vi "HideHistoryGraph.vi"(8 "error in":errorcluster caption="错误输入（无错误）", 11 "PCM MenuVIPanelSplit.lvclass":refnum<class "PCM MenuVIPanelSplit.lvclass">) -> (0 "error out":errorcluster caption="错误输出", 3 "PCM MenuVIPanelSplit.lvclass out":refnum<class "PCM MenuVIPanelSplit.lvclass">)   [LabVIEW 2016, in "PCM MenuVIPanelSplit.lvclass"]
uses:
  PCM MenuVIPanelSplit.lvclass
  C:/Users/CL/Desktop/ZcDAQprj0811/ZcDAQprj/Modules/DAQ-Display/PanelSplitToolkit/PanelRootNode/PanelRootNode.lvclass
  PanelSplitToolkit/PanelRootNode/PanelRootNode.lvclass
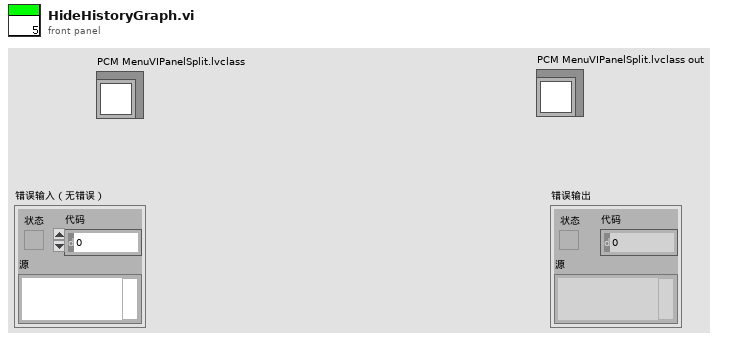
[diagram p1: front panel]
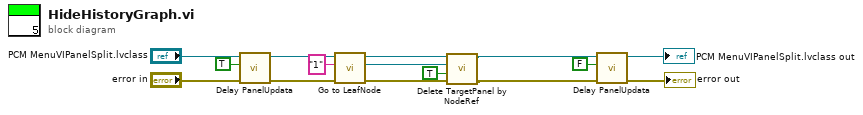
[diagram p0: block diagram]
diagram:
  n1 = call "Delay PanelUpdata.vi"("error in"="error in", "延迟前面板更新"=TRUE, "PanelRootNode 输入"="PCM MenuVIPanelSplit.lvclass") -> ("error out"=w13:errorcluster, "PanelRootNode 输出"=w11:refnum<class "PCM MenuVIPanelSplit.lvclass">)  [unwired: 7 in]
  n2 = call-dynamic "Go to LeafNode.vi"("error in"=w13, "LeafNumber"="1", "PanelRootNode 输入"=w11) -> ("error out"=w4:errorcluster, "Node*"=w2:refnum<data-value>, "PanelRootNode 输出"=w6:refnum<class "PCM MenuVIPanelSplit.lvclass">)  [unwired: 5 in, 1 out]
  n3 = call-dynamic "Delete TargetPanel by NodeRef.vi"("error in"=w4, "Abort VI"=TRUE, "Node*"=w2, "PanelRootNode 输入"=w6) -> ("error out"=w3:errorcluster, "PanelRootNode 输出"=w5:refnum<class "PCM MenuVIPanelSplit.lvclass">)  [unwired: 6 in]
  n4 = call "Delay PanelUpdata.vi"("error in"=w3, "延迟前面板更新"=FALSE, "PanelRootNode 输入"=w5) -> ("error out"=→"error out":errorcluster, "PanelRootNode 输出"=→"PCM MenuVIPanelSplit.lvclass out":refnum<class "PCM MenuVIPanelSplit.lvclass">)  [unwired: 7 in]
